vi "Refresh Listbox.vi"(11 "ListboxBusMonitorPanel in":refnum<class "ListboxBusMonitorPanel.lvclass">) -> (3 "ListboxBusMonitorPanel out":refnum<class "ListboxBusMonitorPanel.lvclass">)   [LabVIEW 2020, in "ListboxBusMonitor.lvlib" / "ListboxBusMonitorPanel.lvclass"]
doc: "刷新列表框"
uses:
  ListboxBusMonitorPanel.lvclass
  ListboxBusMonitorPanel.lvclass/ListboxBusMonitorPanel.ctl
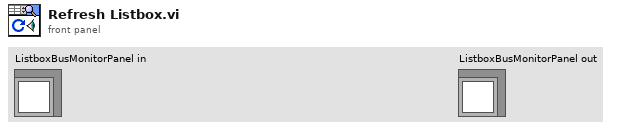
[diagram p1: front panel]
types:
  T1 = cluster{"U64 Count":u64, "Name":string, "Type":string, "Value":string, "Publication Time":string, "Count":string}
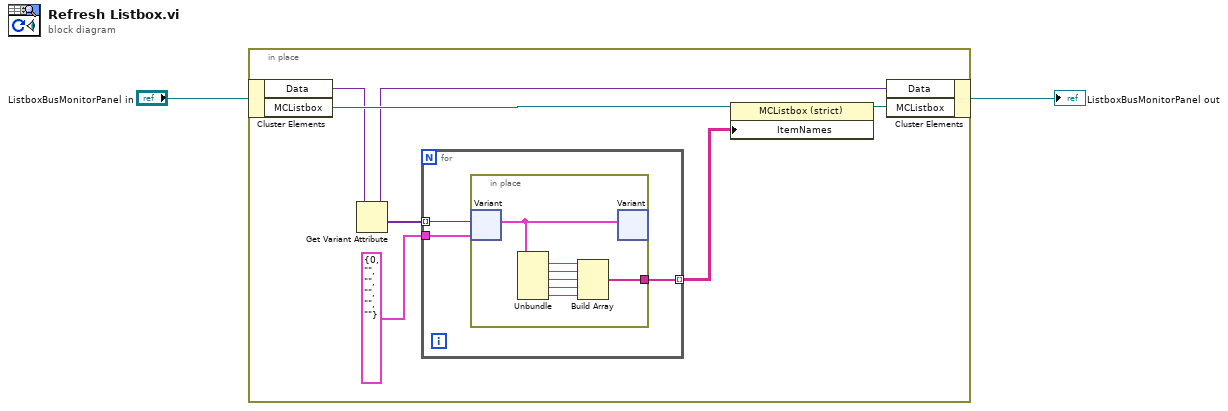
[diagram p0: block diagram]
diagram:
  n1 = in-place {
    n2 = in-place-cluster #1("ListboxBusMonitorPanel in") -> ("Data"=w7:variant, "MCListbox"=w9:refnum<vi>)
    n3 = Get Variant Attribute(Variant=w7) -> (duplicate Variant=w6:variant, values=w5:variant[])  [unwired: 3 in, 2 out]
    n4 = for {
      tunnel: w5 -> [w12] mode=indexing
      tunnel: T1 {"U64 Count"=0, "Name"="", "Type"="", "Value"="", "Publication Time"="", "Count"=""} -> [w11]
      tunnel: [w10] -> w3 mode=indexing
      n5 = in-place {
        in-place-border: [w18] -> w10
        n6 = in-place-variant #2(w12, w11) -> (w19:T1)  [unwired: 1 out]
        n7 = Unbundle(w19) -> ("Name"=w17:string, "Type"=w16:string, "Value"=w15:string, "Publication Time"=w14:string, "Count"=w13:string)  [unwired: 1 out]
        n8 = Build Array(w17, w16, w15, w14, w13) -> (w18:string[])
        n9 = in-place-variant #2(w19) -> ()  [unwired: 2 out]
      }
    }
    n10 = property class="MCListbox (strict)"(reference=w9, "ItemNames"=w3) -> (reference out=w8:refnum<vi>)  [unwired: 1 in, 1 out]
    n11 = in-place-cluster #1("Data"=w6, "MCListbox"=w8) -> (→"ListboxBusMonitorPanel out":refnum<class "ListboxBusMonitorPanel.lvclass">)
  }
